vi "NeutralZone.vi"(9 "Alliance":enum16{"Blue", "Red"}(ring), 10 "Gear Side":enum16{"Center", "Left", "Right"}(ring), 11 "RobotDriveDevRef":T1={"DevStatus"={"status"=FALSE, "code"=0, "source"=""}, "Motors[]"=[], "Square Inputs"=FALSE, "Max Output"=1.0}) -> (3 "RobotDriveDevRef 2":T1={"DevStatus"={"status"=FALSE, "code"=0, "source"=""}, "Motors[]"=[], "Square Inputs"=FALSE, "Max Output"=1.0})   [LabVIEW 2016]
uses:
  <vilib>/Rock Robotics/WPI/RobotDrive/WPI_RobotDriveDevRef.ctl
  <vilib>/Rock Robotics/WPI/MotorControl/WPI_MotorControlDeviceRef.ctl
  <vilib>/Rock Robotics/WPI/MotorControl/WPI_MotorControlType.ctl
  <vilib>/Rock Robotics/SystemInterfaces/DIO/FPGA_DIOPWMChannel.ctl
  <vilib>/Rock Robotics/WPI/PWM/WPI_PWMDeadband.ctl
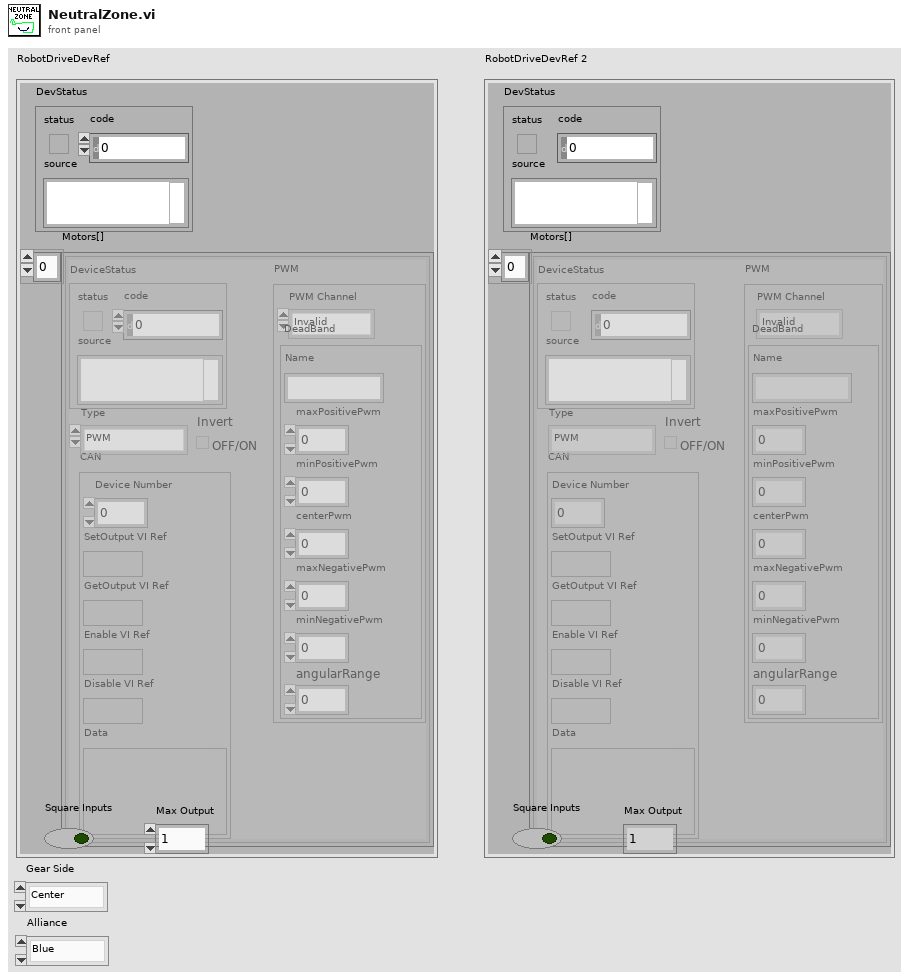
[diagram p1: front panel]
types:
  T1 = typedef "WPI_RobotDriveDevRef.ctl" = cluster{"DevStatus":errorcluster, "Motors[]":T2[], "Square Inputs":bool, "Max Output":dbl}
  T2 = typedef "WPI_MotorControlDeviceRef.ctl" = cluster{"DeviceStatus":errorcluster, "Type":T3, "PWM":cluster{"PWM Channel":T4, "DeadBand":T5}, "CAN":cluster{"Device Number":u8, "SetOutput VI Ref":variant, "GetOutput VI Ref":variant, "Enable VI Ref":variant, "Disable VI Ref":variant, "Data":variant}, "Invert":bool}
  T3 = typedef "WPI_MotorControlType.ctl" = enum16{"PWM", "CAN"}
  T4 = typedef "FPGA_DIOPWMChannel.ctl" = enum8{"PWM 0", "PWM 1", "PWM 2", "PWM 3", "PWM 4", "PWM 5", "PWM 6", "PWM 7", "PWM 8", "PWM 9", "PWM MXP 0", "PWM MXP 1", "PWM MXP 2", "PWM MXP 3", "PWM MXP 4", "PWM MXP 5", "PWM MXP 6", "PWM MXP 7", "PWM MXP 8", "PWM MXP 9", "Invalid"}
  T5 = typedef "WPI_PWMDeadband.ctl" = cluster{"Name":string, "maxPositivePwm":i32, "minPositivePwm":i32, "centerPwm":i32, "maxNegativePwm":i32, "minNegativePwm":i32, "angularRange":u16}
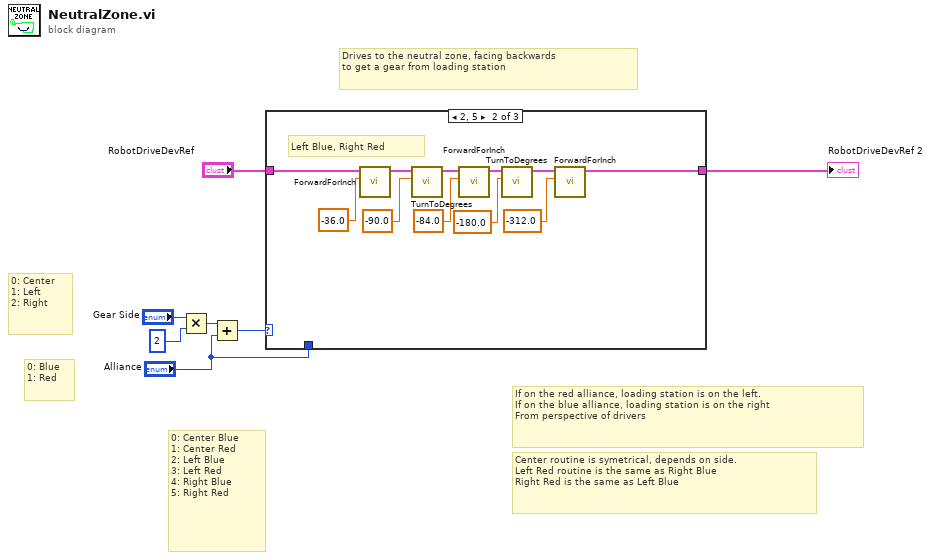
[diagram p0: block diagram]
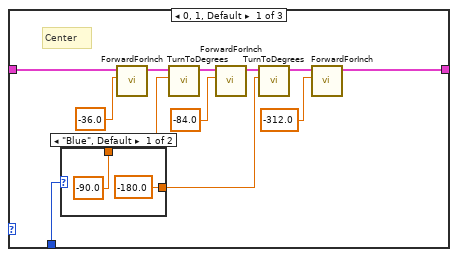
[diagram p2: hidden frame]
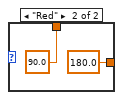
[diagram p3: hidden frame]
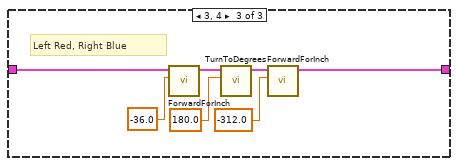
[diagram p4: hidden frame]
diagram:
  # "Drives to the neutral zone, facing backwards\nto get a gear from loading station"
  # "0: Center Blue\n1: Center Red\n2: Left Blue\n3: Left Red\n4: Right Blue\n5: Right Red"
  # "0: Blue\n1: Red"
  # "0: Center\n1: Left\n2: Right"
  # "Center routine is symetrical, depends on side.\nLeft Red routine is the same as Right Blue\nRight Red is the same as Left Blue"
  # "If on the red alliance, loading station is on the left.\nIf on the blue alliance, loading station is on the right\nFrom perspective of drivers"
  n1 = Multiply(x="Gear Side", y=2) -> (x*y=w6:i32)
  n2 = Add(x=w6, y="Alliance") -> (x+y=w3:i32)
  n3 = case shown="2, 5" w3 {
    tunnel: "RobotDriveDevRef" -> [w12 w25 w35]
    tunnel: [w11 w24 w36] -> w2
    tunnel: "Alliance" -> [w10 _ _]
    frame 0, 1, Default {
      # "Center"
      n4 = case shown="\"Blue\", Default" w10 {
        tunnel: [-180.0 ("Distance") 180.0 ("Distance")] -> w9
        tunnel: [-90.0 ("Distance") 90.0 ("Distance")] -> w8
        frame "Blue", Default {
        }
        frame "Red" {
        }
      }
      n5 = call "ForwardForInch.vi"("Distance"=-36.0, "RobotDriveDevRef"=w12) -> ("RobotDriveDevRef 2"=w18:T1)  [unwired: 9 in]
      n6 = call "TurnToDegrees.vi"("Angle"=w8, "RobotDriveDevRef"=w18) -> ("RobotDriveDevRef 2"=w17:T1)  [unwired: 9 in]
      n7 = call "ForwardForInch.vi"("Distance"=-84.0, "RobotDriveDevRef"=w17) -> ("RobotDriveDevRef 2"=w15:T1)  [unwired: 9 in]
      n8 = call "TurnToDegrees.vi"("Angle"=w9, "RobotDriveDevRef"=w15) -> ("RobotDriveDevRef 2"=w14:T1)  [unwired: 9 in]
      n9 = call "ForwardForInch.vi"("Distance"=-312.0, "RobotDriveDevRef"=w14) -> ("RobotDriveDevRef 2"=w11:T1)  [unwired: 9 in]
    }
    frame 2, 5 {
      # "Left Blue, Right Red"
      n10 = call "ForwardForInch.vi"("Distance"=-36.0, "RobotDriveDevRef"=w25) -> ("RobotDriveDevRef 2"=w27:T1)  [unwired: 9 in]
      n11 = call "TurnToDegrees.vi"("Angle"=-90.0 ("Distance"), "RobotDriveDevRef"=w27) -> ("RobotDriveDevRef 2"=w29:T1)  [unwired: 9 in]
      n12 = call "ForwardForInch.vi"("Distance"=-84.0, "RobotDriveDevRef"=w29) -> ("RobotDriveDevRef 2"=w31:T1)  [unwired: 9 in]
      n13 = call "TurnToDegrees.vi"("Angle"=-180.0 ("Distance"), "RobotDriveDevRef"=w31) -> ("RobotDriveDevRef 2"=w33:T1)  [unwired: 9 in]
      n14 = call "ForwardForInch.vi"("Distance"=-312.0, "RobotDriveDevRef"=w33) -> ("RobotDriveDevRef 2"=w24:T1)  [unwired: 9 in]
    }
    frame 3, 4 {
      # "Left Red, Right Blue"
      n15 = call "ForwardForInch.vi"("Distance"=-36.0, "RobotDriveDevRef"=w35) -> ("RobotDriveDevRef 2"=w40:T1)  [unwired: 9 in]
      n16 = call "TurnToDegrees.vi"("Angle"=180.0 ("Distance"), "RobotDriveDevRef"=w40) -> ("RobotDriveDevRef 2"=w38:T1)  [unwired: 9 in]
      n17 = call "ForwardForInch.vi"("Distance"=-312.0, "RobotDriveDevRef"=w38) -> ("RobotDriveDevRef 2"=w36:T1)  [unwired: 9 in]
    }
  }
  "RobotDriveDevRef 2" <- w2
